vi "练习2-自动扫频.vi"   [LabVIEW 2021]
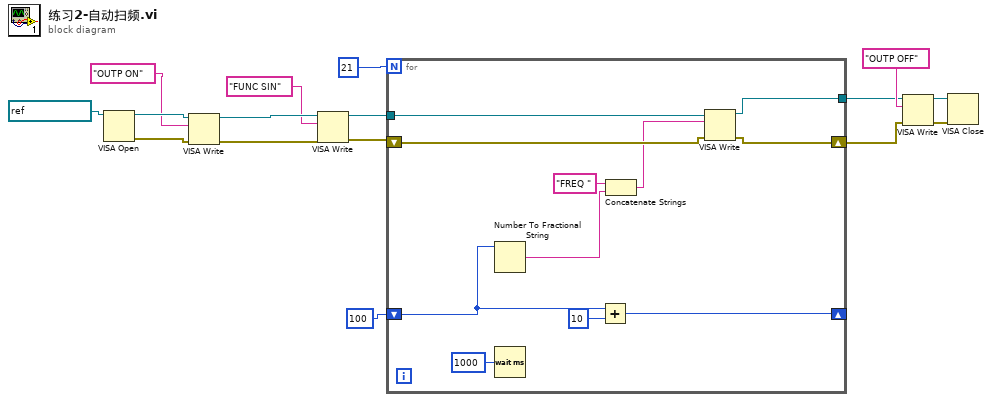
[diagram p0: block diagram]
diagram:
  n1 = VISA Open(VISA resource name=refnum<visa-resource-name> "DG1022U") -> (VISA resource name=w15:refnum<visa-resource-name>, error out=w14:errorcluster)  [unwired: 4 in]
  n2 = VISA Write(VISA resource name=w15, write buffer="OUTP ON", error in (no error)=w14) -> (VISA resource name out=w12:refnum<visa-resource-name>, error out=w10:errorcluster)  [unwired: 1 out]
  n3 = VISA Write(VISA resource name=w12, write buffer="FUNC SIN", error in (no error)=w10) -> (VISA resource name out=w5:refnum<visa-resource-name>, error out=w3:errorcluster)  [unwired: 1 out]
  n4 = for {
    N: 21 -> [_]
    tunnel: w5 -> [w27]
    tunnel: [w26] -> w4
    shift-right: [w24] -> w2
    shift-left: w3 -> [w25]
    shift-right: [w18] -> _
    shift-left: 100 -> [w20]
    n5 = Number To Fractional String(number=w20) -> (F-format string=w21:string)  [unwired: 3 in]
    n6 = Wait (ms)(milliseconds to wait=u32 1000) -> ()  [unwired: 1 out]
    n7 = Add(x=w20, y=10) -> (x+y=w18:i32)
    n8 = Concatenate Strings("FREQ " ("string"), w21) -> (w23:string)
    n9 = VISA Write(VISA resource name=w27, write buffer=w23, error in (no error)=w25) -> (VISA resource name out=w26:refnum<visa-resource-name>, error out=w24:errorcluster)  [unwired: 1 out]
  }
  n10 = VISA Write(VISA resource name=w4, write buffer="OUTP OFF", error in (no error)=w2) -> (VISA resource name out=w7:refnum<visa-resource-name>, error out=w8:errorcluster)  [unwired: 1 out]
  n11 = VISA Close(VISA resource name=w7, error in (no error)=w8) -> ()  [unwired: 1 out]
